vi "Time-Y Circ Buffer.vi"(9 "buffer [1024]":i32=1024, 10 "Y in":dbl[](array[numeric]), 11 "XY in":cluster{timestamp[], dbl[]}[](array[cluster])) -> (3 "XY":cluster{timestamp[], dbl[]}[](array[cluster]))   [LabVIEW 2019, in "Instrument UI.Temperhum.lvclass"]
uses:
  Instrument UI.Temperhum/Instrument UI.Temperhum.lvclass
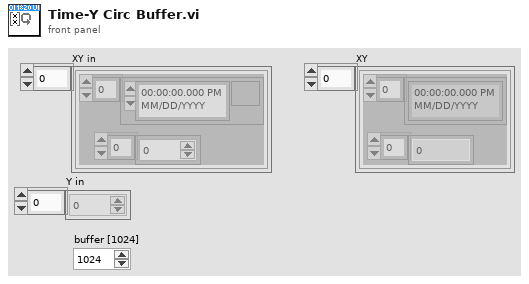
[diagram p1: front panel]
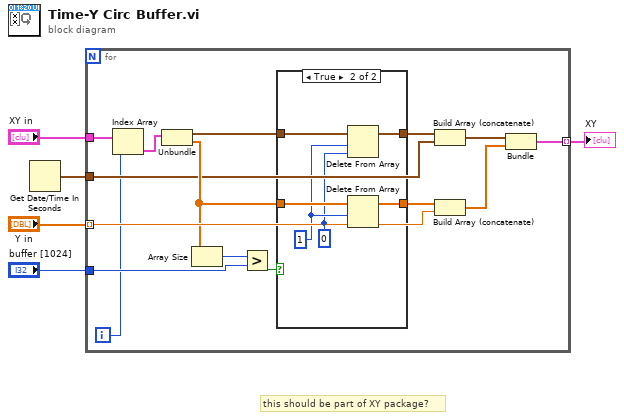
[diagram p0: block diagram]
diagram:
  # "this should be part of XY package?"
  n1 = Get Date/Time In Seconds() -> (seconds since 1Jan1904=w1:timestamp)
  n2 = for {
    tunnel: "buffer [1024]" -> [w20]
    tunnel: "Y in" -> [w19] mode=indexing
    tunnel: [w18] -> w3 mode=indexing
    tunnel: "XY in" -> [w8]
    tunnel: w1 -> [w9]
    i -> [w6]
    n3 = Index Array(array=w8, index=w6) -> (element=w7:cluster{timestamp[], dbl[]})
    n4 = Unbundle(w7) -> (w12:timestamp[], w11:dbl[])
    n5 = Array Size(array=w11) -> (size(s)=w16:i32)
    n6 = Greater?(x=w16, y=w20) -> (0:w13:bool)
    n7 = case shown="True" w13 {
      tunnel: w11 -> [w22 w28]
      tunnel: [w22 w27] -> w15
      tunnel: w12 -> [w21 w25]
      tunnel: [w21 w24] -> w14
      frame False {
      }
      frame True {
        w23 = 0 ("length")
        w26 = 1 ("length")
        n8 = Delete From Array(array=w25, length=w26, index=w23) -> (array with subset deleted=w24:timestamp[])  [unwired: 1 out]
        n9 = Delete From Array(array=w28, length=w26, index=w23) -> (array with subset deleted=w27:dbl[])  [unwired: 1 out]
      }
    }
    n10 = Build Array (concatenate)(w14, w9) -> (w17:timestamp[])
    n11 = Build Array (concatenate)(w15, w19) -> (w10:dbl[])
    n12 = Bundle(w17, w10) -> (w18:cluster{timestamp[], dbl[]})  [unwired: 1 in]
  }
  "XY" <- w3
